vi "Write IP.vi"(8 "error in (no error)":errorcluster, 10 "IP":string, 11 "Ini File in":refnum<class "Ini File.lvclass">) -> (0 "error out":errorcluster, 3 "Ini File out":refnum<class "Ini File.lvclass">)   [LabVIEW 2025, in "File Library.lvlib" / "Ini File.lvclass"]
uses:
  Ini File.lvclass
  Ini File.lvclass/Ini File.ctl
  <vilib>/Utility/config.llb/Write Key (String).vi
  <vilib>/Utility/config.llb/NI_LVConfig.lvlib
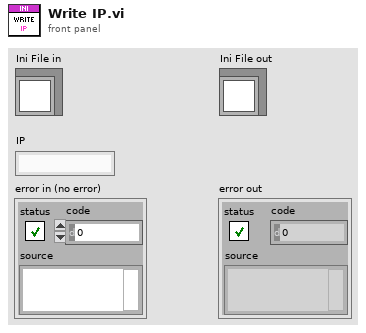
[diagram p1: front panel]
types:
  T1 = typedef "NI_LVConfig.lvlib/Config Data RefNum.ctl" = refnum<k1>
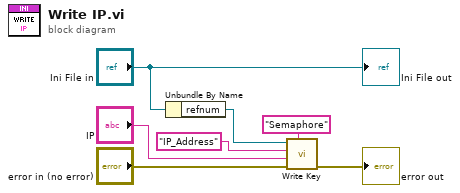
[diagram p0: block diagram]
diagram:
  n1 = Unbundle By Name("Ini File in") -> ("refnum"=w4:T1)
  n2 = call-poly <vilib>:"Write Key.vi"("section"="Semaphore", "error in (no error)"="error in (no error)", "value"="IP", "key"="IP_Address" ("section"), "refnum"=w4) -> ("error out"=→"error out":errorcluster)  [unwired: 4 in, 2 out]
  "Ini File out" <- "Ini File in"
